vi "Append Image to Report (path).vi"(0 "report in":refnum<class "ooCalc.lvclass">, 1 "alignment (default)":T1, 2 "MS Office parameters":T2, 7 "path or URL of image":path, 9 "caption or alternative string":string, 11 "error in (no error)":errorcluster) -> (4 "report out":refnum<class "ooCalc.lvclass">, 8 "start out (Word)":i32, 10 "end out (Word)":i32, 15 "error out":errorcluster)   [LabVIEW 2009, in "ooCalc.lvclass"]
doc: "For an HTML report, the VI embeds a link to an image into the report. For a standard report, the VI appends the image from a file. You can wire either a path to the image or a string that contains the image URL to this polymorphic VI. The data type you wire to the <B>path or URL of image</B> input determines the polymorphic instance to use."
uses:
  ooCalc.lvclass
  <vilib>/Utility/NIReport.llb/HTML Report Image Alignment.ctl
  C:/Projets/LAVAG/OpenOfficeRGT/AODL/DLLs/AODL.dll
  ooCalc.lvclass/ooCalc.ctl
  <vilib>/Utility/NIReport.llb/NI_ReportGenerationCore.lvlib
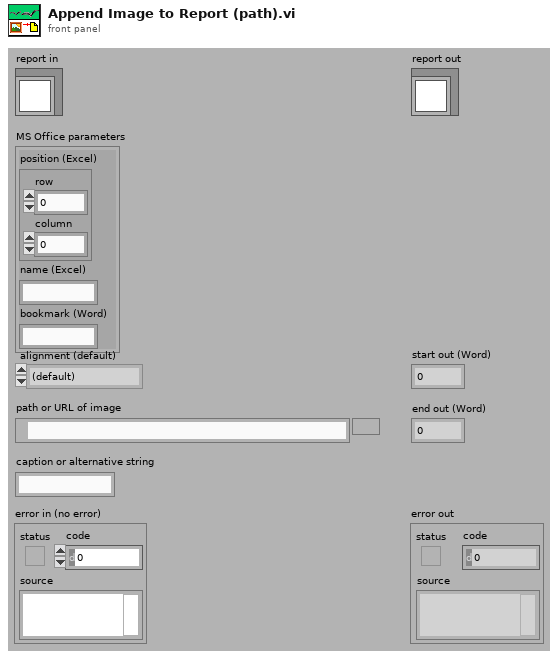
[diagram p1: front panel]
types:
  T1 = typedef "NI_ReportGenerationCore.lvlib/HTML Report Image Alignment.ctl" = enum16{"(default)", "LEFT", "RIGHT", "TOP", "TEXTTOP", "MIDDLE", "ABSMIDDLE", "BASELINE", "BOTTOM", "ABSBOTTOM"}
  T2 = cluster{"position (Excel)":cluster{"row":i32, "column":i32}, "name (Excel)":string, "bookmark (Word)":string}
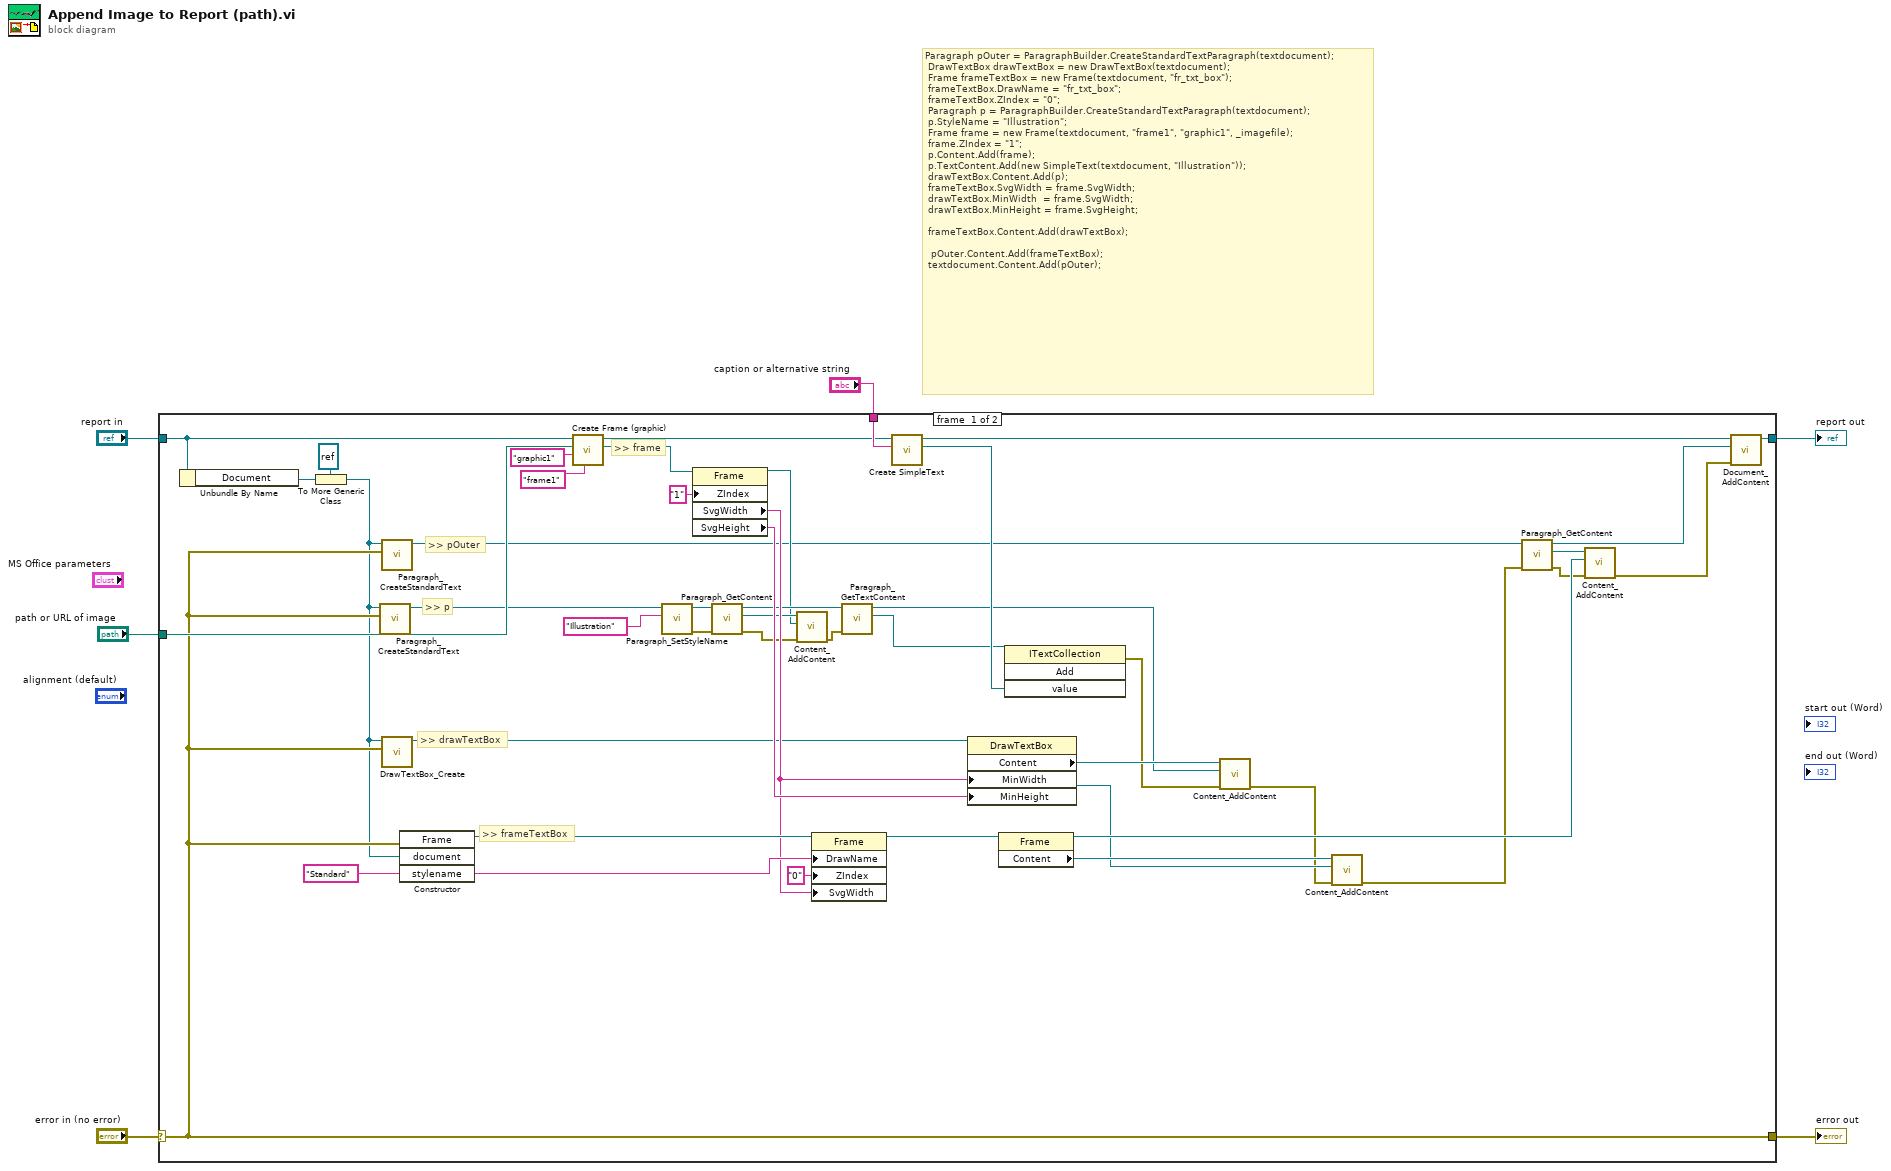
[diagram p0: block diagram]
diagram:
  # "Paragraph pOuter = ParagraphBuilder.CreateStandardTextParagraph(textdocument);\n DrawTextBox drawTextBox = new DrawTextBox(textdocument);\n Frame frameTextBox = new Frame(textdocument, \"fr_txt_box\");\n frameTextBox.DrawName = \"fr_txt_box\";\n frameTextBox.ZIndex = \"0\";\n Paragraph p = ParagraphBuilder.CreateStandardTextParagraph(textdocument);\n p.StyleName = \"Illustration\";\n Frame frame = new Frame(textdocument, \"frame1\", \"graphic1\", _imagefile);\n frame.ZIndex = \"1\";\n p.Content.Add(frame);\n p.TextContent.Add(new SimpleText(textdocument, \"Illustration\"));\n drawTextBox.Content.Add(p);\n frameTextBox.SvgWidth = frame.SvgWidth;\n drawTextBox.MinWidth  = frame.SvgWidth;\n drawTextBox.MinHeight = frame.SvgHeight;\n\n frameTextBox.Content.Add(drawTextBox);\n\n  pOuter.Content.Add(frameTextBox);\n textdocument.Content.Add(pOuter);"
  n1 = case shown="No Error" "error in (no error)" {
    selector: "error in (no error)" -> [w12 w52]
    tunnel: [w12 w52] -> w5
    tunnel: "report in" -> [w18 w53]
    tunnel: [w51 w53] -> w3
    tunnel: "path or URL of image" -> [w46 _]
    tunnel: "caption or alternative string" -> [w37 _]
    frame #0 {
      w49 = "Standard" ("frameStyleName")
      # ">> frame"
      # ">> p"
      # ">> frameTextBox"
      # ">> drawTextBox"
      # ">> pOuter"
      n2 = Unbundle By Name(w18) -> ("Document"=w9:refnum<k24>)
      n3 = To More Generic Class(target class=refnum<k24> refnum, reference=w9) -> (generic class reference=w8:refnum<k24>)
      n4 = call "Paragraph_CreateStandardText.vi"("error in"=w12, "document"=w8) -> ("StandardTextParagraph"=w19:refnum<k24>)  [unwired: 8 in, 1 out]
      n5 = call "Paragraph_CreateStandardText.vi"("error in"=w12, "document"=w8) -> ("StandardTextParagraph"=w17:refnum<k24>)  [unwired: 8 in, 1 out]
      n6 = call "DrawTextBox_Create.vi"("error in"=w12, "document"=w8) -> ("DrawTextBox"=w11:refnum<k24>)  [unwired: 8 in, 1 out]
      n7 = constructor class="Frame"(error in=w12, "document"=w8, "stylename"=w49) -> (reference out=w50:refnum<k24>)  [unwired: 2 in, 4 out]
      n8 = call-dynamic "Create Frame (graphic).vi"("stylename"="frame1", "drawName"="graphic1", "Graphic file"=w46, "ooWriter in"=w18) -> ("Frame (graphic)"=w42:refnum<k24>, "ooWriter out"=w7:refnum<class "ooCalc.lvclass">)  [unwired: 5 in, 1 out]
      n9 = call "Paragraph_SetStyleName.vi"("StyleName"="Illustration", "Paragraph"=w19) -> ("error out"=w30:errorcluster, "Paragraph dup"=w34:refnum<k24>)  [unwired: 8 in]
      n10 = property class="Frame"(reference=w42, "ZIndex"="1") -> (reference out=w31:refnum<k24>, "SvgWidth"=w40:string, "SvgHeight"=w41:string)  [unwired: 1 in, 1 out]
      n11 = call "Paragraph_GetContent.vi"("error in"=w30, "Paragraph"=w34) -> ("error out"=w28:errorcluster, "ContentCollection"=w32:refnum<k24>, "Paragraph dup"=w36:refnum<k24>)  [unwired: 7 in]
      n12 = call "Content_AddContent.vi"("error in"=w28, "Content"=w31, "ContentCollection"=w32) -> ("error out"=w29:errorcluster)  [unwired: 7 in, 1 out]
      n13 = property class="Frame"(reference=w50, "DrawName"=w49, "ZIndex"="0", "SvgWidth"=w40) -> (reference out=w47:refnum<k24>)  [unwired: 1 in, 1 out]
      n14 = call "Paragraph_GetTextContent.vi"("error in"=w29, "Paragraph"=w36) -> ("TextContent Collection"=w35:refnum<k24>, "Paragraph dup"=w23:refnum<k24>)  [unwired: 7 in, 1 out]
      n15 = call-dynamic "Create SimpleText.vi"("simpleText"=w37, "ooDocument"=w7) -> ("SimpleText"=w38:refnum<k24>, "ooDocument out"=w39:refnum<class "ooCalc.lvclass">)  [unwired: 7 in, 1 out]
      n16 = property class="DrawTextBox"(reference=w11, "MinWidth"=w40, "MinHeight"=w41) -> (reference out=w21:refnum<k24>, "Content"=w25:refnum<k24>)  [unwired: 1 in, 1 out]
      n17 = property class="Frame"(reference=w47) -> (reference out=w27:refnum<k24>, "Content"=w22:refnum<k24>)  [unwired: 1 in, 1 out]
      n18 = invoke class="ITextCollection" method="Add"(reference=w35, "value"=w38) -> (error out=w24:errorcluster)  [unwired: 2 in, 3 out]
      n19 = call "Content_AddContent.vi"("error in"=w24, "Content"=w23, "ContentCollection"=w25) -> ("error out"=w20:errorcluster)  [unwired: 7 in, 1 out]
      n20 = call "Content_AddContent.vi"("error in"=w20, "Content"=w21, "ContentCollection"=w22) -> ("error out"=w13:errorcluster)  [unwired: 7 in, 1 out]
      n21 = call "Paragraph_GetContent.vi"("error in"=w13, "Paragraph"=w17) -> ("error out"=w14:errorcluster, "ContentCollection"=w15:refnum<k24>, "Paragraph dup"=w16:refnum<k24>)  [unwired: 7 in]
      n22 = call "Content_AddContent.vi"("error in"=w14, "Content"=w27, "ContentCollection"=w15) -> ("error out"=w26:errorcluster)  [unwired: 7 in, 1 out]
      n23 = call-dynamic "Document_AddContent.vi"("error in (no error)"=w26, "Content"=w16, "ooWriter in"=w39) -> ("ooWriter out"=w51:refnum<class "ooCalc.lvclass">)  [unwired: 7 in, 1 out]
    }
    frame #1 {
    }
  }
  "error out" <- w5
  "report out" <- w3
